vi "11-1.vi"() -> ()   [LabVIEW 2022 SP3, in "AoC22.lvlib"]
uses:
  AoC22.lvlib
  Monkey/Worry Level.ctl
  011b0bfd-92be-469c-bd34-b9fef4f027b3.vi
  <vilib>/Comparison/Less/Less Functor/Less Functor.lvclass
  Monkey/Monkey.lvclass
panel:
  out "Insp":u64[](array[numeric])
  out "Round":i32
  out "old":T1
  out "string array":string[](array[string])
  out "Monkey Business":u64
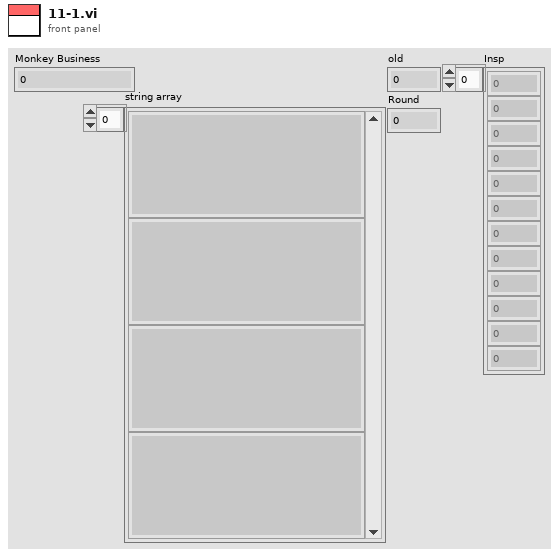
[diagram p1: front panel]
types:
  T1 = typedef "AoC22.lvlib/Monkey.lvclass/Worry Level.ctl" = u64
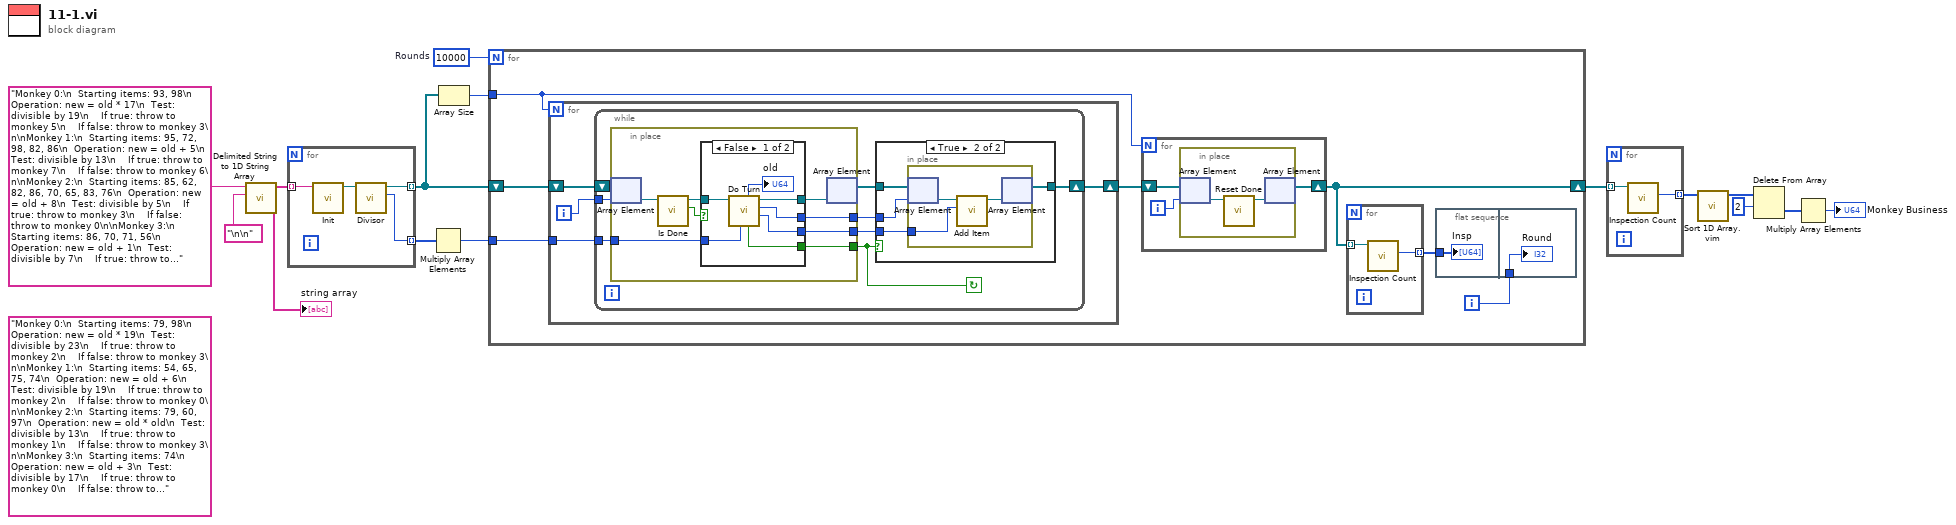
[diagram p0: block diagram]
diagram:
  (unwired) "Monkey 0:\n  Starting items: 79, 98\n  Operation: new = old * 19\n  Test: divisible by 23\n    If true: throw to monkey 2\n    If false: throw to monkey 3\n\nMonkey 1:\n  Starting items: 54, 65, 75, 74\n  Operation: new = old + 6\n  Test: divisible by 19\n    If true: throw to monkey 2\n    If false: throw to monkey 0\n\nMonkey 2:\n  Starting items: 79, 60, 97\n  Operation: new = old * old\n  Test: divisible by 13\n    If true: throw to monkey 1\n    If false: throw to monkey 3\n\nMonkey 3:\n  Starting items: 74\n  Operation: new = old + 3\n  Test: divisible by 17\n    If true: throw to monkey 0\n    If false: throw to monkey 1"
  w12 = 10000  # Rounds
  n1 = call <vilib>:"Delimited String to 1D String Array.vi"("delimiter"="\n\n", "delimited string"="Monkey 0:\n  Starting items: 93, 98\n  Operation: new = old * 17\n  Test: divisible by 19\n    If true: throw to monkey 5\n    If false: throw to monkey 3\n\nMonkey 1:\n  Starting items: 95, 72, 98, 82, 86\n  Operation: new = old + 5\n  Test: divisible by 13\n    If true: throw to monkey 7\n    If false: throw to monkey 6\n\nMonkey 2:\n  Starting items: 85, 62, 82, 86, 70, 65, 83, 76\n  Operation: new = old + 8\n  Test: divisible by 5\n    If true: throw to monkey 3\n    If false: throw to monkey 0\n\nMonkey 3:\n  Starting items: 86, 70, 71, 56\n  Operation: new = old + 1\n  Test: divisible by 7\n    If true: throw to monkey 4\n    If false: throw to monkey 5\n\nMonkey 4:\n  Starting items: 77, 71, 86, 52, 81, 67\n  Operation: new = old + 4\n  Test: divisible by 17\n    If true: throw to monkey 1\n    If false: throw to monkey 6\n\nMonkey 5:\n  Starting items: 89, 87, 60, 78, 54, 77, 98\n  Operation: new = old * 7\n  Test: divisible by 2\n    If true: throw to monkey 1\n    If false: throw to monkey 4\n\nMonkey 6:\n  Starting items: 69, 65, 63\n  Operation: new = old + 6\n  Test: divisible by 3\n    If true: throw to monkey 7\n    If false: throw to monkey 2\n\nMonkey 7:\n  Starting items: 89\n  Operation: new = old * old\n  Test: divisible by 11\n    If true: throw to monkey 0\n    If false: throw to monkey 2") -> ("string array"=w13:string[])  [unwired: 9 in]
  "string array" <- w13
  n2 = for {
    tunnel: w13 -> [w18] mode=indexing
    tunnel: [w16] -> w11 mode=indexing
    tunnel: [w15] -> w3 mode=indexing
    n3 = call "Init.vi"("Input"=w18) -> ("Monkey"=w17:refnum<class "Monkey.lvclass">)  [unwired: 10 in]
    n4 = call "Divisor.vi"("Monkey in"=w17) -> ("Div Test"=w15:T1, "Monkey out"=w16:refnum<class "Monkey.lvclass">)  [unwired: 8 in, 1 out]
  }
  n5 = Multiply Array Elements(1:w3) -> (0:w2:T1)
  n6 = Array Size(array=w11) -> (size(s)=w10:i32)
  n7 = for {
    N: w12 -> [_]
    shift-right: [w22] -> w9
    shift-left: w11 -> [w25]
    tunnel: w10 -> [w24]
    tunnel: w2 -> [w19]
    i -> [w20]
    n8 = for {
      N: w24 -> [_]
      shift-right: [w36] -> w23
      shift-left: w25 -> [w38]
      tunnel: w19 -> [w35]
      i -> [w37]
      n9 = while {
        tunnel: w37 -> [w45]
        shift-right: [w41] -> w36
        shift-left: w38 -> [w46]
        tunnel: w35 -> [w39]
        stop <- w40 continue-if-true
        n10 = in-place {
          in-place-border: [w58] -> w44
          in-place-border: [w57] -> w42
          in-place-border: [w56] -> w40
          in-place-border: w39 -> [w55]
          n11 = in-place-array #1(w46, w45) -> (w62:refnum<class "Monkey.lvclass">)
          n12 = call "Is Done.vi"("Monkey in"=w62) -> ("Is Done?"=w61:bool, "Monkey out"=w60:refnum<class "Monkey.lvclass">)  [unwired: 8 in, 1 out]
          n13 = case shown="False" w61 {
            tunnel: w60 -> [w69 w70]
            tunnel: [w68 w70] -> w59
            tunnel: [w67 _] -> w58
            tunnel: [w66 _] -> w57
            tunnel: [w65 _] -> w56
            tunnel: w55 -> [w63 _]
            frame False {
              n14 = call "Do Turn.vi"("Divisor"=w63, "Monkey in"=w69) -> ("Item"=w66:T1, "Dest"=w67:i32, "Monkey out"=w68:refnum<class "Monkey.lvclass">, "Throw?"=w65:bool, "old"=→"old":T1)  [unwired: 4 in, 1 out]
            }
            frame True {
            }
          }
          n15 = in-place-array #1(w59) -> (w43:refnum<class "Monkey.lvclass">[])  [unwired: 1 out]
        }
        n16 = case shown="True" w40 {
          tunnel: w44 -> [_ w51]
          tunnel: w43 -> [w47 w50]
          tunnel: w42 -> [_ w49]
          tunnel: [w47 w48] -> w41
          frame False {
          }
          frame True {
            n17 = in-place {
              in-place-border: w49 -> [w52]
              n18 = in-place-array #2(w50, w51) -> (w54:refnum<class "Monkey.lvclass">)
              n19 = call "Add Item.vi"("Item"=w52, "Monkey in"=w54) -> ("Monkey out"=w53:refnum<class "Monkey.lvclass">)  [unwired: 8 in, 1 out]
              n20 = in-place-array #2(w53) -> (w48:refnum<class "Monkey.lvclass">[])  [unwired: 1 out]
            }
          }
        }
      }
    }
    n21 = for {
      N: w24 -> [_]
      shift-right: [w31] -> w22
      shift-left: w23 -> [w32]
      i -> [w30]
      n22 = in-place {
        n23 = in-place-array #3(w32, w30) -> (w34:refnum<class "Monkey.lvclass">)
        n24 = call "Reset Done.vi"("Monkey in"=w34) -> ("Monkey out"=w33:refnum<class "Monkey.lvclass">)  [unwired: 9 in, 1 out]
        n25 = in-place-array #3(w33) -> (w31:refnum<class "Monkey.lvclass">[])  [unwired: 1 out]
      }
    }
    n26 = for {
      tunnel: w22 -> [w29] mode=indexing
      tunnel: [w28] -> w21 mode=indexing
      n27 = call "Inspection Count.vi"("Monkey in"=w29) -> ("Inspections"=w28:u64)  [unwired: 8 in, 2 out]
    }
    n28 = flat-sequence {
      tunnel: w21 -> [w26]
      tunnel: w20 -> [w27]
      frame #0 {
        "Insp" <- w26
      }
      frame #1 {
        "Round" <- w27
      }
    }
  }
  n29 = for {
    tunnel: w9 -> [w72] mode=indexing
    tunnel: [w71] -> w8 mode=indexing
    n30 = call "Inspection Count.vi"("Monkey in"=w72) -> ("Inspections"=w71:u64)  [unwired: 8 in, 2 out]
  }
  n31 = call "Sort 1D Array.vim"("unsorted array"=w8) -> ("sorted array"=w7:u64[])  [unwired: 10 in]
  n32 = Delete From Array(array=w7, length=2) -> (deleted portion=w5:u64[])  [unwired: 1 in, 1 out]
  n33 = Multiply Array Elements(1:w5) -> (0:→"Monkey Business":u64)
